vi "Kill All Tasks.vi"() -> ()   [LabVIEW 2015, in "Reaper.lvclass"]
uses:
  Reaper.lvclass
  Reaper.lvclass/Reaper.ctl
panel:
  out "standard output":string[](array[string])
  out "cmd string":string
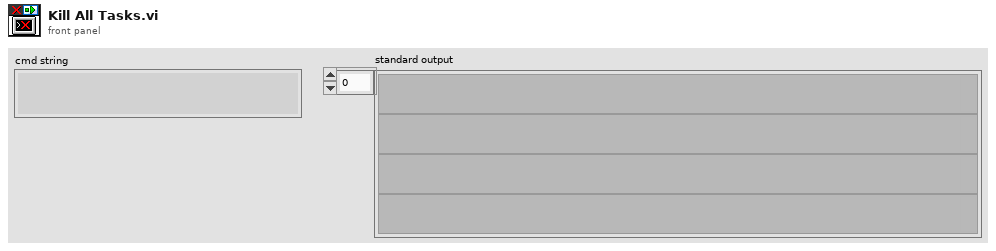
[diagram p1: front panel]
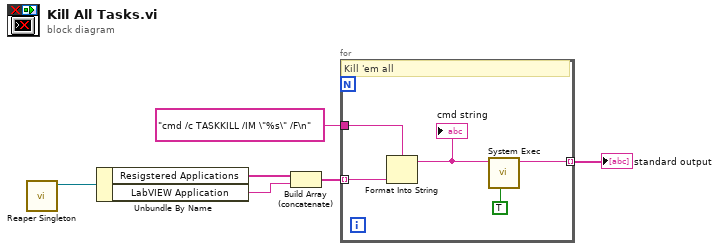
[diagram p0: block diagram]
diagram:
  n1 = call "Reaper Singleton.vi"() -> ("Reaper Out"=w6:refnum<class "Reaper.lvclass">)  [unwired: 11 in]
  n2 = Unbundle By Name(w6) -> ("Resigstered Applications"=w2:string[], "LabVIEW Application"=w1:string)
  n3 = Build Array (concatenate)(w2, w1) -> (w4:string[])
  n4 = for {
    tunnel: w4 -> [w7] mode=indexing
    tunnel: "cmd /c TASKKILL /IM \"%s\" /F\n" ("format string") -> [w11]
    tunnel: [w9] -> w3 mode=indexing
    # "Kill 'em all"
    n5 = Format Into String(format string=w11, w7) -> (resulting string=w10:string)  [unwired: 2 in, 1 out]
    "cmd string" <- w10
    n6 = call <vilib>:"System Exec.vi"("run minimized? (F)"=TRUE, "command line"=w10) -> ("standard output"=w9:string)  [unwired: 6 in, 3 out]
  }
  "standard output" <- w3
